vi "Level Meter.vi"() -> ()   [LabVIEW 2009, in "Magnet.lvclass"]
uses:
  Magnet.lvclass
  Oxford/BUSGEN.LLB/OxfordAddress.ctl
panel:
  in  "ILM Setup":T2={"Address"={"Com Port"=1, "ISOBUS Address"=5, "GPIB Address"=24, "Communication"=enum."ISOBUS"}, "ILM Name"="", "Display Channel"=[]}
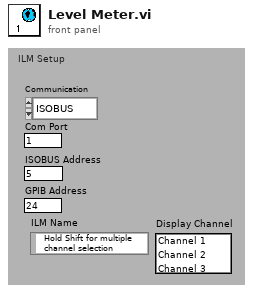
[diagram p1: front panel]
types:
  T1 = typedef "OxfordAddress.ctl" = cluster{"Com Port":i32, "ISOBUS Address":i32, "GPIB Address":i16, "Communication":enum16{"RS232", "ISOBUS", "GPIB", "Gateway"}}
  T2 = cluster{"Address":T1, "ILM Name":string, "Display Channel":i32[]}
diagram:
